vi "Front Camera Circle detect.vi"() -> ()   [LabVIEW 2014]
uses:
  <vilib>/vision/Shape Detection.llb/ShapeDetectionMatchOptions.ctl
  <vilib>/vision/Pattern Matching.llb/IMAQ Match Range Setting.ctl
  <vilib>/vision/Pattern Matching.llb/IMAQ Curve Parameters.ctl
  Global.vi
  <vilib>/vision/NI_Vision_Development_Module.lvlib
panel:
  out "Score":dbl
  out "Number of Matches Returned":i32
  in  "Curve Parameters":T1={"Extraction Mode"=0, "Edge Threshold"=150, "Edge Filter Size"=1, "Min Length"=25, "Row Search Step Size"=15, "Col Search Step Size"=15, "Max Endpoint Gap"=10, "Closed"=TRUE, "Subpixel"=FALSE} {"Extraction Mode" items=["Normal", "Uniform Regions"]; "Edge Filter Size" items=["Fine", "Normal", "Contour Tracing"]; "Max Endpoint Gap" min=0; "Col Search Step Size" min=1 max=255 step=1; "Row Search Step Size" min=1 max=255 step=1; "Min Length" min=0; "Edge Threshold" min=1 max=350 step=1}
  out "error out":errorcluster
  in  "Minimum match score":dbl=900.0
  in  "Match Options":T2={"Rotation"=FALSE, "Scale"=FALSE, "Occlusion"=TRUE, "Range Settings"=[{"Match Constraints"=0, "Min"=0.0, "Max"=0.0}, {"Match Constraints"=1, "Min"=0.0, "Max"=0.0}, {"Match Constraints"=2, "Min"=0.0, "Max"=25.0}]} {"Range Settings"."Max" format="%.2f"; "Range Settings"."Min" format="%.2f"; "Range Settings"."Match Constraints" items=["Rotation Angle (degrees)", "Scale Factor (%)", "Occlusion (%)"]}
  in  "Circle Descriptor":cluster{"Min Radius":dbl, "Max Radius":dbl}={"Min Radius"=20.0, "Max Radius"=400.0}
  out "Image":T4(plugin-control)
  in  "stop video":bool
  in  "milliseconds to wait":u32
  out "Read Video":errorcluster
  out "x-y":u32=19
  # "Range"
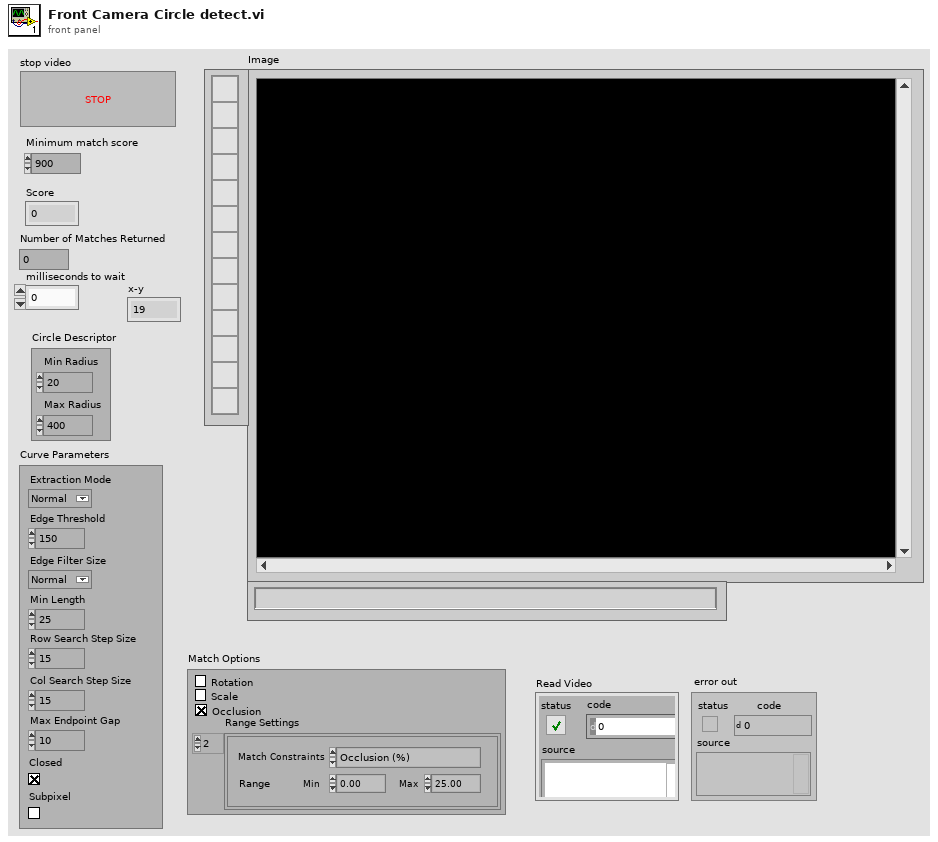
[diagram p1: front panel]
types:
  T1 = typedef "IMAQ Curve Parameters.ctl" = cluster{"Extraction Mode":u32, "Edge Threshold":i32, "Edge Filter Size":u32, "Min Length":i32, "Row Search Step Size":i32, "Col Search Step Size":i32, "Max Endpoint Gap":i32, "Closed":bool, "Subpixel":bool}
  T2 = typedef "ShapeDetectionMatchOptions.ctl" = cluster{"Rotation":bool, "Scale":bool, "Occlusion":bool, "Range Settings":T3[]}
  T3 = typedef "IMAQ Match Range Setting.ctl" = cluster{"Match Constraints":u32, "Min":dbl, "Max":dbl}
  T4 = typedef "IMAQ Image.ctl" = refnum<image>
  T5 = typedef "Image Type" = u32
  T6 = cluster{"Position":cluster{"X":sgl, "Y":sgl}, "Radius":dbl, "Score":dbl}[]
  T7 = cluster{"Position":cluster{"X":sgl, "Y":sgl}, "Radius":dbl, "Score":dbl}
  T8 = cluster{"Left":i32, "Top":i32, "Right":i32, "Bottom":i32}
  T9 = typedef "Control cluster.ctl" = cluster{"Roll":sgl, "Pitch":sgl, "Vertical Speed":sgl, "Yaw Speed":sgl}
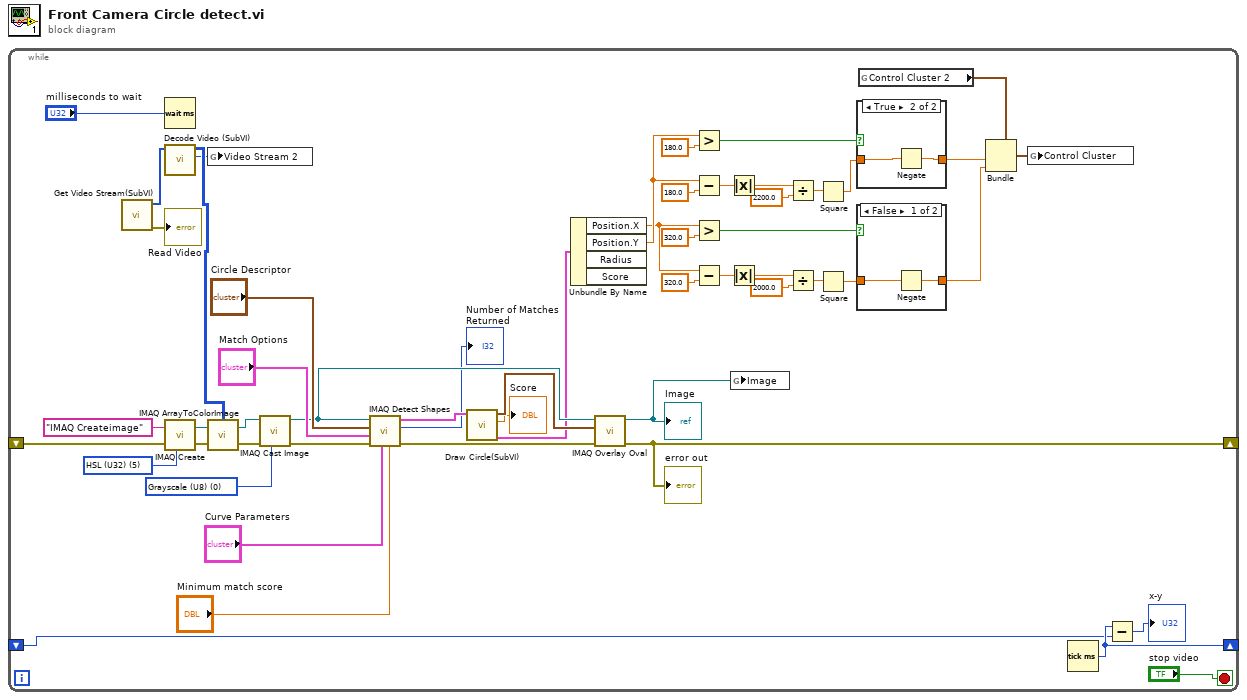
[diagram p0: block diagram]
diagram:
  n1 = while {
    shift-right: [w44] -> _
    shift-left: _ -> [w43]
    shift-right: [w29] -> _
    shift-left: _ -> [w40]
    stop <- "stop video" stop-if-true
    w37 = T5 0 items=["Grayscale (U8)", "Grayscale (I16)", "Grayscale (SGL)", "Complex (CSG)", "RGB (U32)", "HSL (U32)", "RGB (U64)", "Grayscale (U16)"] ("Image Type")
    w50 = T5 5 items=["Grayscale (U8)", "Grayscale (I16)", "Grayscale (SGL)", "Complex (CSG)", "RGB (U32)", "HSL (U32)", "RGB (U64)", "Grayscale (U16)"] ("Image Type")
    n2 = call "Get Video Stream(SubVI).vi"() -> ("error out"=→"Read Video":errorcluster, "ImgData"=w51:u8[])  [unwired: 10 in]
    n3 = Wait (ms)(milliseconds to wait="milliseconds to wait") -> ()  [unwired: 1 out]
    n4 = call "Decode Video (SubVI).vi"("ImgData"=w51) -> ("new picture"=w41:picture, "Array"=w47:u32[][])  [unwired: 9 in]
    n5 = call "IMAQ Create"("Image Name"="IMAQ Createimage", "Image Type"=w50, "error in (no error)"=w40) -> ("New Image"=w46:T4, "error out"=w45:errorcluster)  [unwired: 2 in]
    n6 = global write "Global.vi" "Video Stream 2"(w41) -> ()
    n7 = call "IMAQ ArrayToColorImage"("Image Pixels (U32)"=w47, "Image"=w46, "error in (no error)"=w45) -> ("Image Out"=w38:T4, "error out"=w39:errorcluster)  [unwired: 2 in]
    n8 = call "IMAQ Cast Image"("Image Type"=w37, "error in (no error)"=w39, "Image Src"=w38) -> ("error out"=w34:errorcluster, "Image Dst Out"=w32:T4)  [unwired: 7 in]
    n9 = call-poly "IMAQ Detect Shapes"("Minimum match score"="Minimum match score", "Curve Parameters"="Curve Parameters", "error in (no error)"=w34, "Match Options"="Match Options", "Circle Descriptor"="Circle Descriptor", "Image"=w32) -> ("error out"=w31:errorcluster, "Number of Matches Returned"=→"Number of Matches Returned":i32, "Circles"=w27:T6)  [unwired: 3 in]
    n10 = call "Draw Circle(SubVI).vi"("Circles"=w27) -> ("element"=w24:T7, "Score"=→"Score":dbl, "Bounding Rectangle out"=w30:T8)  [unwired: 8 in]
    n11 = Unbundle By Name(w24) -> ("Position.X"=w6:sgl, "Position.Y"=w11:sgl)  [unwired: 2 out]
    n12 = call "IMAQ Overlay Oval"("error in (no error)"=w31, "Bounding Rectangle"=w30, "Image"=w32) -> ("error out"=w29:errorcluster, "Image Out"=w22:T4)  [unwired: 7 in]
    "Image" <- w22
    "error out" <- w29
    n13 = Greater?(x=w11, y=180.0) -> (0:w19:bool)
    n14 = Subtract(x=w11, y=180.0) -> (x-y=w14:dbl)
    n15 = Greater?(x=w6, y=320.0) -> (0:w21:bool)
    n16 = Subtract(x=w6, y=320.0) -> (x-y=w9:dbl)
    n17 = Absolute Value(x=w14) -> (abs(x)=w13:dbl)
    n18 = Absolute Value(x=w9) -> (abs(x)=w8:dbl)
    n19 = global write "Global.vi" "Image"(w22) -> ()
    n20 = Divide(x=w13, y=2200.0) -> (x/y=w2:dbl)
    n21 = Divide(x=w8, y=2000.0) -> (x/y=w4:dbl)
    n22 = Square(x=w2) -> (x^2=w3:dbl)
    n23 = Square(x=w4) -> (x^2=w5:dbl)
    n24 = case shown="True" w19 {
      tunnel: w3 -> [w57 w59]
      tunnel: [w57 w58] -> w16
      frame False {
      }
      frame True {
        n25 = Negate(x=w59) -> (-x=w58:dbl)
      }
    }
    n26 = case shown="False" w21 {
      tunnel: w5 -> [w55 w56]
      tunnel: [w54 w56] -> w17
      frame False {
        n27 = Negate(x=w55) -> (-x=w54:dbl)
      }
      frame True {
      }
    }
    n28 = global read "Global.vi" "Control Cluster 2"() -> (w1:T9)
    n29 = Bundle(cluster=w1, "Vertical Speed"=w16, "Yaw Speed"=w17) -> (w23:T9)  [unwired: 2 in]
    n30 = global write "Global.vi" "Control Cluster"(w23) -> ()
    n31 = Tick Count (ms)() -> (millisecond timer value=w44:u32)
    n32 = Subtract(x=w44, y=w43) -> (x-y=→"x-y":u32)
  }
